vi "daqhat_tcp_scan.vi"(8 "error in (no error)":errorcluster, 9 "Sample count":u32, 10 "Analog channel":u8, 11 "TCP network connection in":refnum<k5>) -> (0 "error out":errorcluster, 1 "Sample data":dbl[](array[numeric]), 2 "Samples read":u32, 3 "TCP Network Connection out":refnum<k5>)   [LabVIEW 2018]
doc: "Read MCC 172 analog data from a TCP server running on a Raspberry Pi. The TCP server program must be running on the Pi, and the TCP connection already opened to the correct IP address and port. Provide the channel number and sample count."
panel:
  out "Status":u8
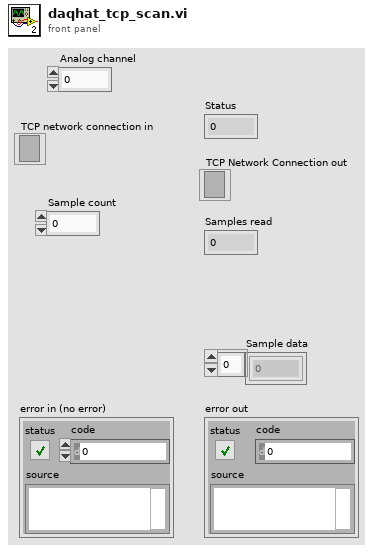
[diagram p1: front panel]
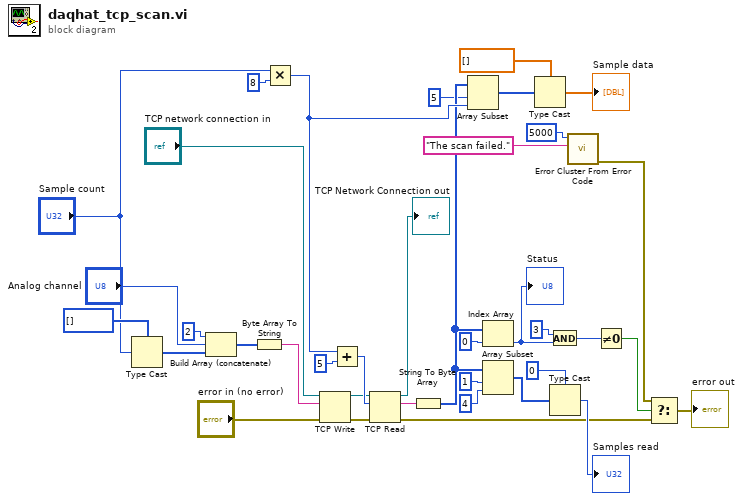
[diagram p0: block diagram]
diagram:
  n1 = Type Cast(type=u8[] [], x="Sample count") -> (*(type *) &x=w18:u8[])
  n2 = Build Array (concatenate)(u8 2, "Analog channel", w18) -> (w25:u8[])
  n3 = Byte Array To String(unsigned byte array=w25) -> (string=w23:string)
  n4 = Multiply(x="Sample count", y=8 ("Sizeof double")) -> (x*y=w37:u32)
  n5 = TCP Write(connection ID="TCP network connection in", data in=w23, error in (no error)="error in (no error)") -> (connection ID out=w20:refnum<k5>, error out=w21:errorcluster)  [unwired: 1 in, 1 out]
  n6 = Add(x=w37, y=5) -> (x+y=w36:u32)
  n7 = TCP Read(connection ID=w20, bytes to read=w36, error in (no error)=w21) -> (connection ID out=→"TCP Network Connection out":refnum<k5>, data out=w22:string, error out=w7:errorcluster)  [unwired: 2 in]
  n8 = String To Byte Array(string=w22) -> (unsigned byte array=w31:u8[])
  n9 = Array Subset(array=w31, index=5, length=w37) -> (w14:u8[])
  n10 = Index Array(array=w31, index=0) -> (element=w4:u8)
  "Status" <- w4
  n11 = Array Subset(array=w31, index=1, length=4) -> (w30:u8[])
  n12 = Type Cast(type=dbl[] [], x=w14) -> (*(type *) &x=→"Sample data":dbl[])
  n13 = And(x=u8 3, y=w4) -> (x .and. y?=w2:u8)
  n14 = Type Cast(type=u32 0, x=w30) -> (*(type *) &x=→"Samples read":u32)
  n15 = call <vilib>:"Error Cluster From Error Code.vi"("error message (\"\")"="The scan failed.", "error code (0)"=5000) -> ("error out"=w6:errorcluster)  [unwired: 7 in]
  n16 = Not Equal To 0?(x=w2) -> (x != 0?=w1:bool)
  n17 = Select(t=w6, s=w1, f=w7) -> (s? t:f=→"error out":errorcluster)
